vi "Modbus Multiple Reads.vi"(8 "Error In":errorcluster, 9 "# elements to read":u16, 10 "Starting Address":u16, 11 "Modbus Master In":refnum<class "Modbus Master.lvclass">) -> (0 "Error Out":errorcluster, 2 "register values":u16[](array[numeric]), 3 "Modbus Master Out":refnum<class "Modbus Master.lvclass">)   [LabVIEW 2014]
uses:
  <vilib>/Modbus/master/Modbus Master.lvclass
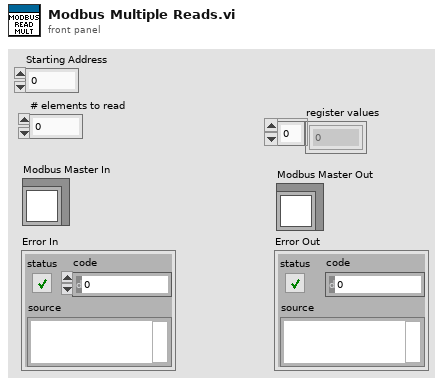
[diagram p1: front panel]
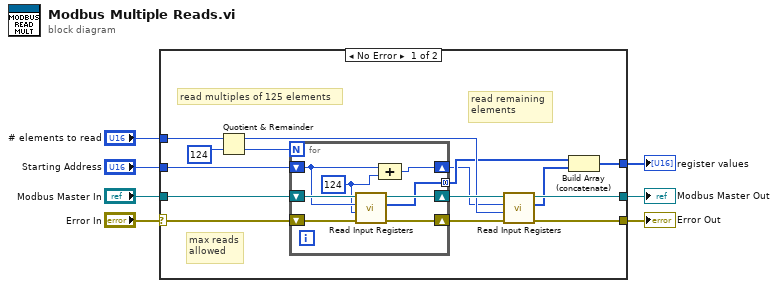
[diagram p0: block diagram]
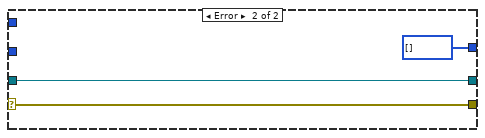
[diagram p2: hidden frame]
diagram:
  n1 = case shown="No Error" "Error In" {
    selector: "Error In" -> [w22 w33]
    tunnel: [w20 w33] -> w6
    tunnel: "Modbus Master In" -> [w19 w32]
    tunnel: [w17 w32] -> w4
    tunnel: "# elements to read" -> [w16 _]
    tunnel: [w12 u16[] []] -> w1
    tunnel: "Starting Address" -> [w9 _]
    frame No Error {
      # "max reads\nallowed"
      # "read remaining\nelements"
      # "read multiples of 125 elements"
      n2 = Quotient & Remainder(x=w16, y=u16 124) -> (x-y*floor(x/y)=w14:u16, floor(x/y)=w8:u16)
      n3 = for {
        N: w8 -> [_]
        shift-right: [w29] -> w21
        shift-left: w22 -> [w30]
        shift-right: [w27] -> w18
        shift-left: w19 -> [w28]
        shift-right: [w24] -> w10
        shift-left: w9 -> [w26]
        tunnel: [w23] -> w11 mode=concatenating
        w25 = u16 124 ("y")
        n4 = call-dynamic "Read Input Registers.vi"("error in (no error)"=w30, "number of input registers"=w25, "starting address"=w26, "Modbus master in"=w28) -> ("error out"=w29:errorcluster, "register values"=w23:u16[], "Modbus master out"=w27:refnum<class "Modbus Master.lvclass">)  [unwired: 5 in]
        n5 = Compound Arithmetic op=ADD(w26, w25) -> (w24:u16)
      }
      n6 = call-dynamic "Read Input Registers.vi"("error in (no error)"=w21, "number of input registers"=w14, "starting address"=w10, "Modbus master in"=w18) -> ("error out"=w20:errorcluster, "register values"=w13:u16[], "Modbus master out"=w17:refnum<class "Modbus Master.lvclass">)  [unwired: 5 in]
      n7 = Build Array (concatenate)(w11, w13) -> (w12:u16[])
    }
    frame Error {
    }
  }
  "Modbus Master Out" <- w4
  "Error Out" <- w6
  "register values" <- w1
